vi "Read Test File.vi"(11 "VI Analyzer in":refnum<class "VI Analyzer.lvclass">) -> (2 "Test File":path)   [LabVIEW 2014, in "VI Analyzer.lvclass"]
uses:
  VI Analyzer.lvclass
  VI Analyzer.lvclass/VI Analyzer.ctl
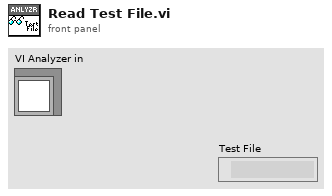
[diagram p1: front panel]
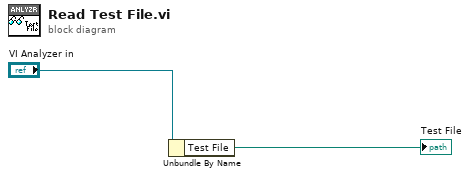
[diagram p0: block diagram]
diagram:
  n1 = Unbundle By Name("VI Analyzer in") -> ("Test File"=→"Test File":path)
